vi "Replacing The Heart - Lesson 7.vi"() -> ()   [LabVIEW 2023]
doc: "This lesson shows that the closures-like co-routines built with channel wires can be established at a higher level diagram than where the co-routine is actually needed, revealing a neat performance advantage that these closure-like functions can have over traditional closure functions."
uses:
  Person Information.ctl
  <extravilib>/ChannelInstances/One Element Stream-t'Person Compare Closure Inputs.ctl'/Read With Abort.vi
  <extravilib>/ChannelInstances/One Element Stream-bool/Write With Abort.vi
  <extravilib>/ChannelInstances/One Element Stream-bool/Instantiate.vi
  <extravilib>/ChannelInstances/One Element Stream-t'Person Compare Closure Inputs.ctl'/Instantiate.vi
  <extravilib>/ChannelInstances/One Element Stream-t'Person Compare Closure Inputs.ctl'/EndpointRead.vi
  <extravilib>/ChannelInstances/One Element Stream-bool/Endpoint.vi
  <extravilib>/ChannelInstances/One Element Stream-t'Person Compare Closure Inputs.ctl'.lvlib
  <extravilib>/ChannelInstances/One Element Stream-bool.lvlib
panel:
  in  "Starting Month":u16(ring) items=["January", "February", "March", "April", "May", "June", "July", "August", "September", "October", "November", "December"]
  in  "Stop":bool
  out "Sorted People":T1[](array[typedef]) {"Birth Date" format="%<%Y/%b/%d>T"}
  in  "Unsorted People":T1[](array[typedef])=[{"ID"=0, "Family Name"="Tennant", "Given Name"="David", "Birth Date"=timestamp(-6434737636.184167 s since 1904-01-01)}, {"ID"=1, "Family Name"="Smith", "Given Name"="Matt", "Birth Date"=timestamp(-6434726400 s since 1904-01-01)}, {"ID"=2, "Family Name"="Li", "Given Name"="Jing", "Birth Date"=timestamp(3091380833.9038334 s since 1904-01-01)}, {"ID"=3, "Family Name"="Patel", "Given Name"="Aadhya", "Birth Date"=timestamp(3093541462.901833 s since 1904-01-01)}, {"ID"=4, "Family Name"="Doe", "Given Name"="Jane", "Birth Date"=timestamp(3154453586.3918333 s since 1904-01-01)}, {"ID"=5, "Family Name"="Rahman", "Given Name"="Mohammed", "Birth Date"=timestamp(3024418078.500833 s since 1904-01-01)}] {"Birth Date" format="%<%Y/%b/%d>T"}
  # "Overview: This lesson shows a variation on the previous lesson.\n\nInstructions:\n1. BEFORE you run the VI, select a Starting Month.\n2. Run the VI. The people will be sorted by birthday but with the people nearest that month prioritized.\n3. Change the Starting Month while the VI is running. Notice that the sort order is unchanged.\n4. Look at the block diagram to see how the sort is done.\n5. Proceed to the next lesson."
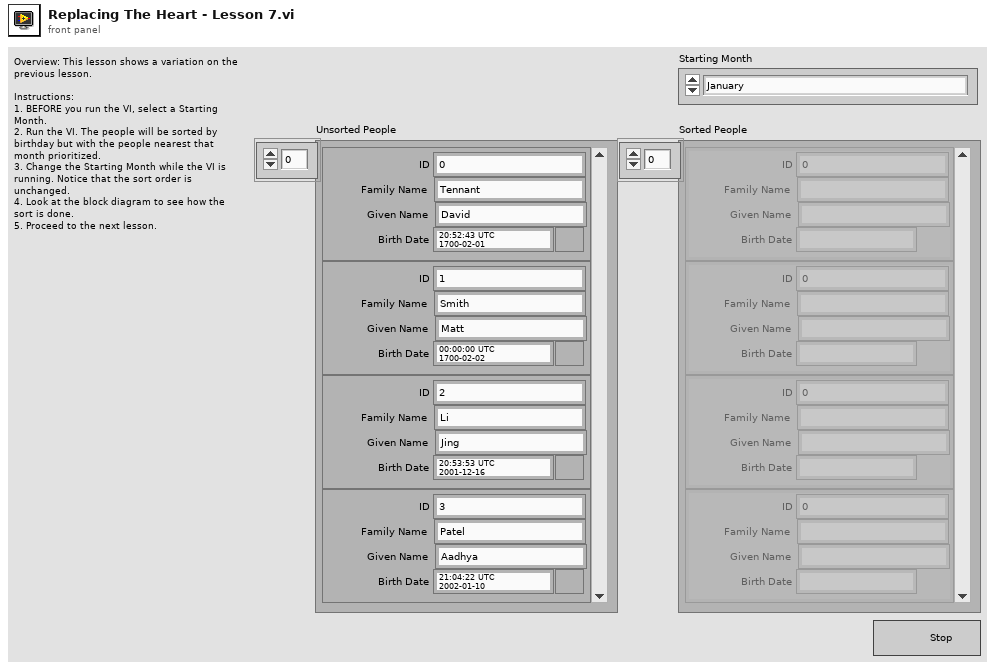
[diagram p1: front panel]
types:
  T1 = typedef "Person Information.ctl" = cluster{"ID":u32, "Family Name":string, "Given Name":string, "Birth Date":timestamp}
  T2 = typedef "One Element Stream-t'Person Compare Closure Inputs.ctl'.lvlib/)Channel.ctl" = refnum<queue>
  T3 = typedef "Person Compare Closure Inputs.ctl" = cluster{"Person A":T1, "Person B":T1}
  T4 = typedef "One Element Stream-bool.lvlib/)Channel.ctl" = refnum<queue>
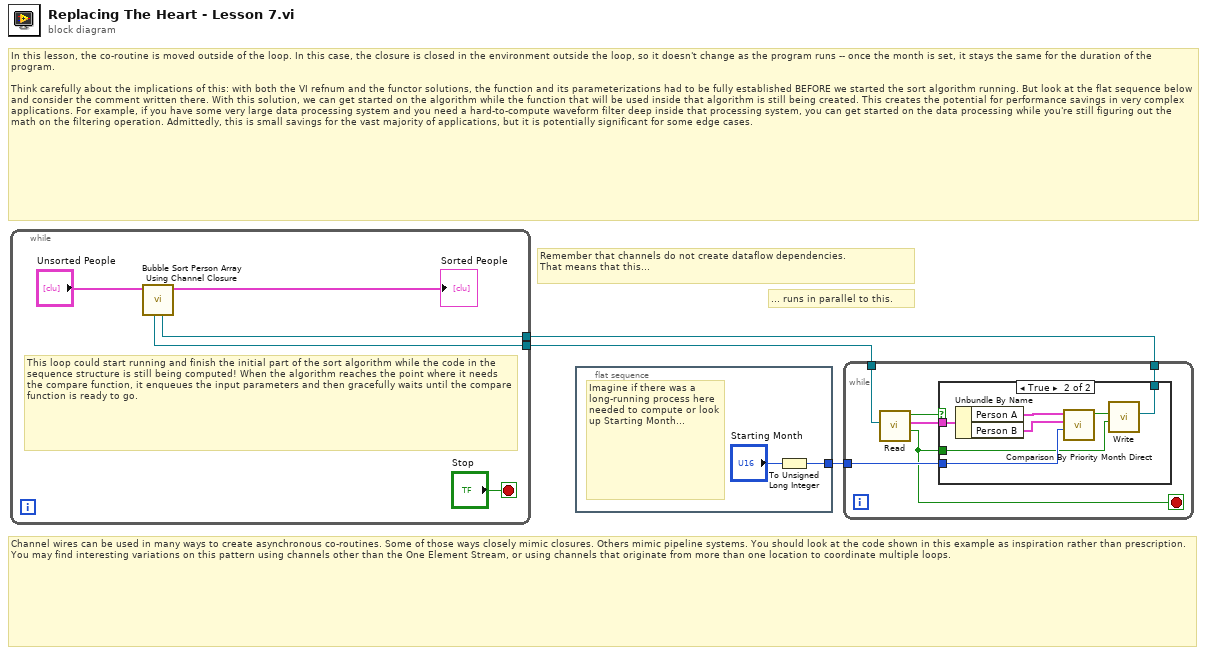
[diagram p0: block diagram]
diagram:
  # "... runs in parallel to this."
  # "Remember that channels do not create dataflow dependencies. \nThat means that this..."
  # "Channel wires can be used in many ways to create asynchronous co-routines. Some of those ways closely mimic closures. Others mimic pipeline systems. You should look at the code shown in this example as inspiration rather than prescription. You may find interesting variations on this pattern using channels other than the One Element Stream, or using channels that originate from more than one location to coordinate multiple loops."
  # "In this lesson, the co-routine is moved outside of the loop. In this case, the closure is closed in the environment outside the loop, so it doesn't change as the program runs -- once the month is set, it stays the same for the duration of the program.\n\nThink carefully about the implications of this: with both the VI refnum and the functor solutions, the function and its parameterizations had to be fully established BEFORE we started the sort algorithm running. But look at the flat sequence below and consider the comment written there. With this solution, we can get started on the algorithm while the function that will be used inside that algorithm is still being created. This creates the potential for performance savings in very complex applications. For example, if you have some very large data processing system and you need a hard-to-compute waveform filter deep inside that processing system, you can get started on the data processing while you're still figuring out the math on the filtering operation. Admittedly, this is small savings for the vast majority of applications, but it is potentially significant for some edge cases."
  n1 = flat-sequence {
    tunnel: [w4] -> w1
    frame #0 {
      # "Imagine if there was a long-running process here needed to compute or look up Starting Month..."
      n2 = To Unsigned Long Integer(number="Starting Month") -> (unsigned 32bit integer=w4:u32)
    }
  }
  n3 = while {
    tunnel: [w7] -> w3
    tunnel: w2 -> [w6]
    stop <- "Stop" stop-if-true
    # "This loop could start running and finish the initial part of the sort algorithm while the code in the sequence structure is still being computed! When the algorithm reaches the point where it needs the compare function, it enqueues the input parameters and then gracefully waits until the compare function is ready to go."
    n4 = call "Bubble Sort Person Array Using Channel Closure.vi"("outputs"=w6, "Unsorted"="Unsorted People") -> ("Sorted"=→"Sorted People":T1[], "inputs"=w7:T2)  [unwired: 8 in]
  }
  n5 = while {
    tunnel: w3 -> [w16]
    tunnel: [w14] -> w2
    tunnel: w1 -> [w12]
    stop <- w11 stop-if-true
    n6 = call <extravilib>:"Read.vi"("channel"=w16) -> ("last element?"=w11:bool, "element"=w15:T3, "element valid?"=w13:bool)  [unwired: 7 in, 1 out]
    n7 = case shown="True" w13 {
      tunnel: w15 -> [_ w23]
      tunnel: [_ w19] -> w14
      tunnel: w12 -> [_ w18]
      tunnel: w11 -> [_ w17]
      frame False {
      }
      frame True {
        n8 = Unbundle By Name(w23) -> ("Person A"=w22:T1, "Person B"=w21:T1)
        n9 = call "Comparison By Priority Month Direct.vi"("Starting Month"=w18, "Person B"=w21, "Person A"=w22) -> ("Swap?"=w20:bool)  [unwired: 8 in]
        n10 = call <extravilib>:"Write.vi"("last element? (F)"=w17, "element"=w20) -> ("channel"=w19:T4)  [unwired: 8 in, 1 out]
      }
    }
  }
